vi "Estimate Pi.vi"(11 "Gamma":dbl[][](array[numeric])) -> (3 "Estimated Pi":dbl[](array[numeric]))   [LabVIEW 2014, in "HMM.lvlib"]
doc: "Estimates the initial state (Pi) with the input HMM model."
uses:
  HMM.lvlib
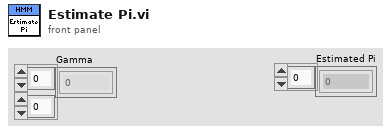
[diagram p1: front panel]
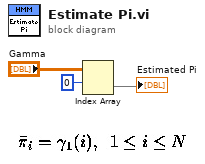
[diagram p0: block diagram]
diagram:
  n1 = Index Array(array="Gamma", index (row)=0) -> (element=→"Estimated Pi":dbl[])  [unwired: 1 in]
